vi "Show_Scrollbars.vi"(8 "error in (no error)":errorcluster, 11 "IB_Tree in":refnum<class "IB_Tree.lvclass">) -> (0 "error out":errorcluster, 3 "IB_Tree out":refnum<class "IB_Tree.lvclass">)   [LabVIEW 2020, in "IB_Tree.lvclass"]
uses:
  <vilib>/AppBuilder/IB_Classes/Tree/IB_Tree.lvclass
  <vilib>/AppBuilder/IB_Classes/Tree/IB_Tree.lvclass/IB_Tree.ctl
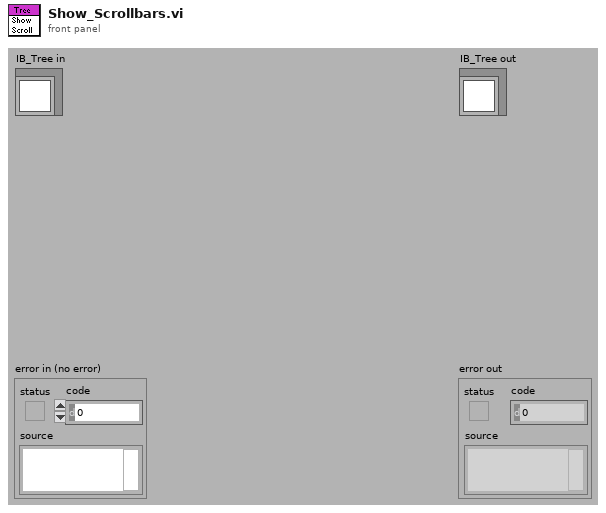
[diagram p1: front panel]
types:
  T1 = typedef "LVNodeAndColumnTypeDef.ctl" = cluster{"Node":string, "Column":i32}
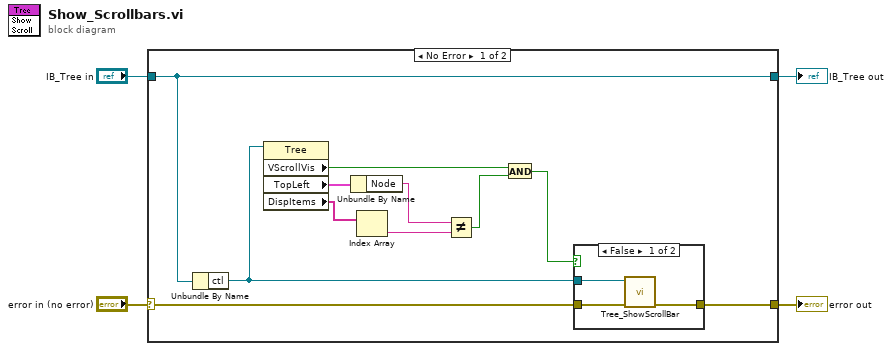
[diagram p0: block diagram]
diagram:
  n1 = case shown="No Error" "error in (no error)" {
    selector: "error in (no error)" -> [w14 w21]
    tunnel: [w13 w21] -> w3
    tunnel: [w15 w20] -> w1
    tunnel: "IB_Tree in" -> [w15 w20]
    frame No Error {
      n2 = Unbundle By Name(w15) -> ("ctl"=w11:refnum<vi>)
      n3 = property class="Tree"(reference=w11) -> ("VScrollVis"=w10:bool, "TopLeft"=w12:T1, "DispItems"=w9:string[])  [unwired: 1 in, 2 out]
      n4 = Unbundle By Name(w12) -> ("Node"=w8:string)
      n5 = Index Array(array=w9) -> (element=w7:string)  [unwired: 1 in]
      n6 = Not Equal?(x=w8, y=w7) -> (x != y?=w6:bool)
      n7 = And(x=w10, y=w6) -> (x .and. y?=w5:bool)
      n8 = case shown="False" w5 {
        tunnel: w14 -> [w18 w19]
        tunnel: [w17 w19] -> w13
        tunnel: w11 -> [w16 _]
        frame False {
          n9 = call <vilib>:"Tree_ShowScrollBar.vi"("error in (no error)"=w18, "Tree"=w16) -> ("error out"=w17:errorcluster)  [unwired: 9 out]
        }
        frame True {
        }
      }
    }
    frame Error {
    }
  }
  "error out" <- w3
  "IB_Tree out" <- w1
